vi "Scanner-PWM_Test.vi"() -> ()   [LabVIEW 2019]
panel:
  in  "Frequency [Hz]":dbl=60.0 format="%#_13g"
  out "Error Out":errorcluster
  in  "Error In":errorcluster
  in  "Stop":bool
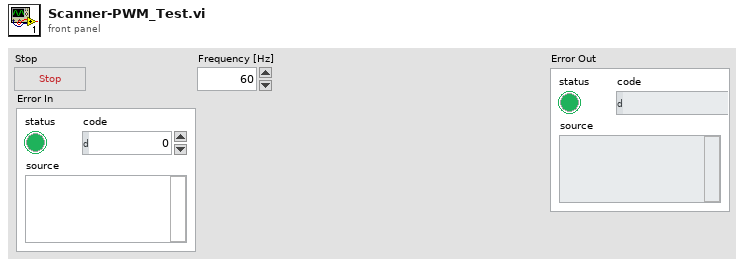
[diagram p1: front panel]
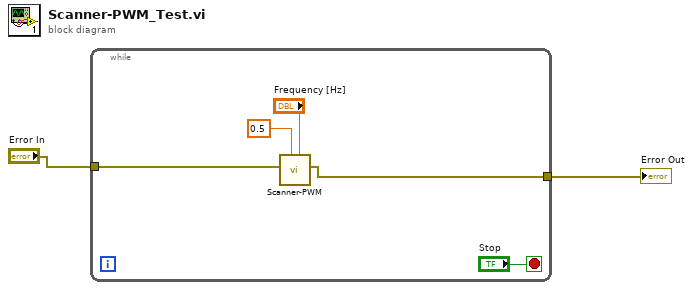
[diagram p0: block diagram]
diagram:
  n1 = while {
    tunnel: "Error In" -> [w6]
    tunnel: [w5] -> w1
    stop <- "Stop" stop-if-true
    n2 = call "Scanner-PWM.vi"("Frequency [Hz]"="Frequency [Hz]", "Duty Cycle"=0.5, "Error In"=w6) -> ("Error Out"=w5:errorcluster)  [unwired: 8 in]
  }
  "Error Out" <- w1
